vi "Get User Interface VI.vi"(8 "error in":errorcluster, 11 "RDMA Transfer Rx User Interface in":refnum<class "RDMA Transfer Rx User Interface.lvclass">=refnum) -> (0 "error out":errorcluster, 2 "user interface vi":refnum<vi>, 3 "RDMA Transfer Rx User Interface out":refnum<class "RDMA Transfer Rx User Interface.lvclass">)   [LabVIEW 2020, in "RDMA.lvlib" / "RDMA Transfer Rx User Interface.lvclass"]
uses:
  RDMA Transfer Rx User Interface.lvclass
  User Interface.vi
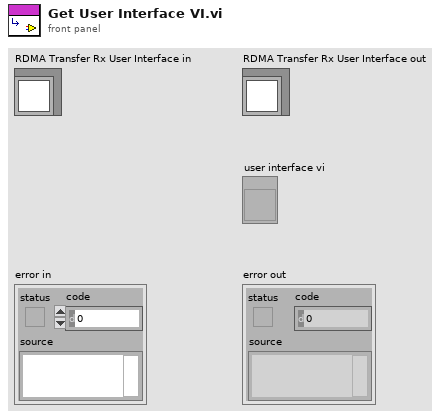
[diagram p1: front panel]
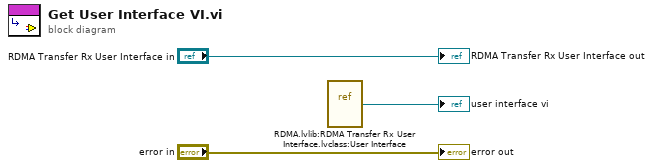
[diagram p0: block diagram]
diagram:
  n1 = vi-ref "RDMA.lvlib:RDMA Transfer Rx User Interface.lvclass:User Interface.vi"() -> (→"user interface vi":refnum<vi>)
  "error out" <- "error in"
  "RDMA Transfer Rx User Interface out" <- "RDMA Transfer Rx User Interface in"
